vi "project to string files.vi"(4 "Export Diagram":bool=TRUE, 6 "Create Captions":bool=TRUE, 8 "error in (no error)":errorcluster, 10 "Project String Files Root":path=path "E:/VI2String/test", 11 "Project Path":path=path "E:/VI2String/Test Project/Test Project.lvproj") -> (0 "error out":errorcluster)   [LabVIEW 2022 SP3]
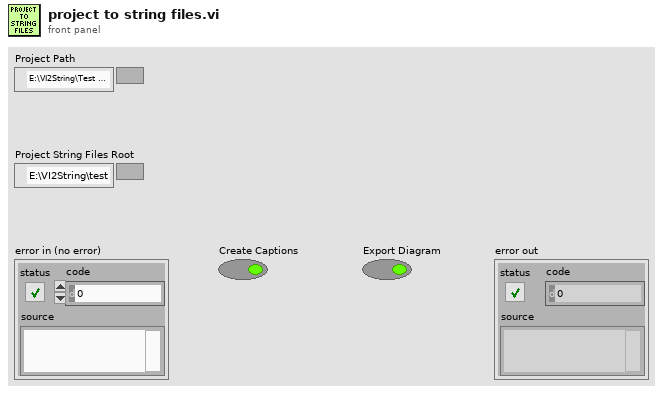
[diagram p1: front panel]
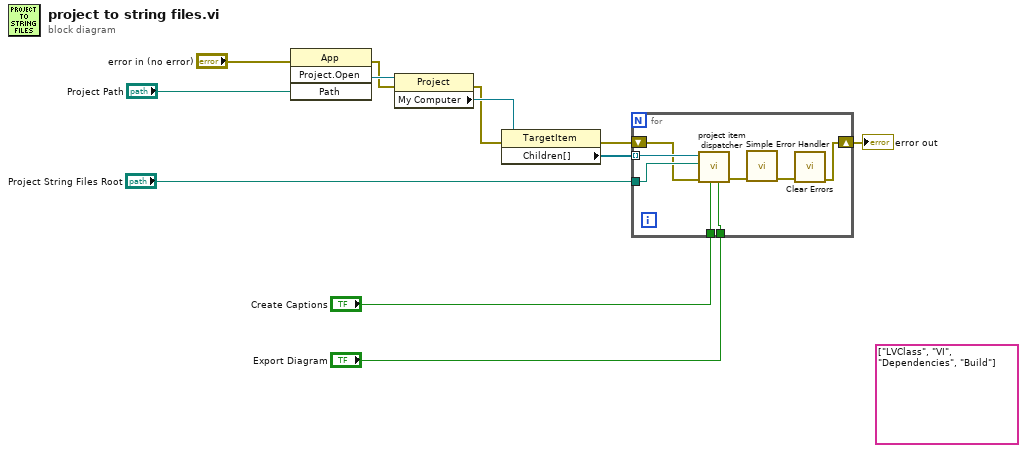
[diagram p0: block diagram]
diagram:
  (unwired) string[] ["LVClass", "VI", "Dependencies", "Build"] ("Array 4")
  n1 = invoke class="App" method="Project.Open"(error in="error in (no error)", "Path"="Project Path") -> (error out=w6:errorcluster, "Project:Open"=w10:refnum<vi>)  [unwired: 2 in, 2 out]
  n2 = property class="Project"(reference=w10, error in=w6) -> (error out=w5:errorcluster, "My Computer"=w11:refnum<vi>)  [unwired: 1 out]
  n3 = property class="TargetItem"(reference=w11, error in=w5) -> (error out=w4:errorcluster, "Children[]"=w12:refnum<vi>[])  [unwired: 1 out]
  n4 = for {
    tunnel: w12 -> [w20] mode=indexing
    tunnel: "Project String Files Root" -> [w19]
    shift-right: [w13] -> w1
    shift-left: w4 -> [w18]
    tunnel: "Create Captions" -> [w17]
    tunnel: "Export Diagram" -> [w16]
    n5 = call "project item dispatcher.vi"("Export Diagram"=w16, "Create Captions"=w17, "error in (no error)"=w18, "String Files Root"=w19, "ProjectItem in"=w20) -> ("error out"=w15:errorcluster)  [unwired: 6 in]
    n6 = call <vilib>:"Simple Error Handler.vi"("error in (no error)"=w15) -> ("error out"=w14:errorcluster)  [unwired: 4 in, 4 out]
    n7 = call <vilib>:"Clear Errors.vi"("error in (no error)"=w14) -> ("error out"=w13:errorcluster)  [unwired: 5 in, 1 out]
  }
  "error out" <- w1
